vi "Find Differences.vi"() -> ()   [LabVIEW 2020]
uses:
  3e53e974-0502-4313-b7b8-032893102bf4.vi
  <vilib>/Utility/file.llb/Read Delimited Spreadsheet (DBL).vi
  <vilib>/Comparison/Equal/Equal Functor/Equal Functor.lvclass
panel:
  out "FrontDelta":dbl
  out "BackDelta":dbl
  out "Redact Data":dbl[][](graph)
  out "Org Data":dbl[][](graph)
  in  "Path":path=path "C:/Amira Data/Strip/Surface_120921_135218.csv"
  # "Average differences between close (compress) and open (decompress)"
  # "(After purging degrading data and 0s)"
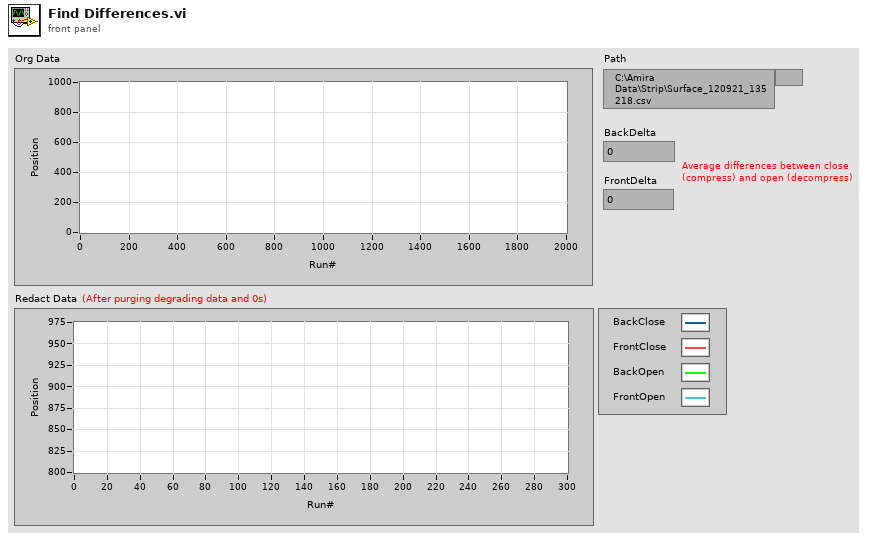
[diagram p1: front panel]
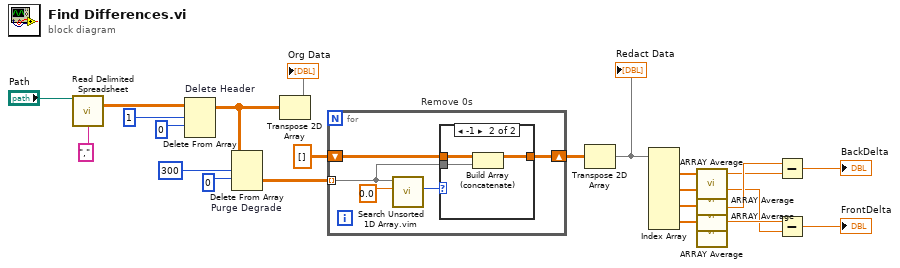
[diagram p0: block diagram]
diagram:
  n1 = call-poly <vilib>:"Read Delimited Spreadsheet.vi"("file path (dialog if empty)"="Path", "delimiter (\\t)"="," ("delimiter (\\t)")) -> ("all rows"=w21:dbl[][])  [unwired: 8 in, 5 out]
  n2 = Delete From Array "Delete Header"(array=w21, length=1, index (row)=0) -> (array with subset deleted=w17:dbl[][])  [unwired: 1 in, 1 out]
  n3 = Delete From Array "Purge Degrade"(array=w17, length=300, index (row)=0) -> (deleted portion=w14:dbl[][])  [unwired: 1 in, 1 out]
  n4 = Transpose 2D Array(2D array=w17) -> (transposed array=→"Org Data":dbl[][])
  n5 = for "Remove 0s" {
    tunnel: w14 -> [w24] mode=indexing
    shift-right: [w25] -> w12
    shift-left: dbl[][] [] -> [w26]
    n6 = call "Search Unsorted 1D Array.vim"("element"=0.0, "unsorted 1D array"=w24) -> ("index of element"=w27:i32)  [unwired: 9 in]
    n7 = case shown="-1" w27 {
      tunnel: w26 -> [w29 w32]
      tunnel: [w29 w31] -> w25
      tunnel: w24 -> [_ w30]
      frame 0, Default {
      }
      frame -1 {
        n8 = Build Array (concatenate)(w32, w30) -> (w31:dbl[][])
      }
    }
  }
  n9 = Transpose 2D Array(2D array=w12) -> (transposed array=w11:dbl[][])
  "Redact Data" <- w11
  n10 = Index Array(array=w11) -> (element #1=w10:dbl[], element #2=w9:dbl[], element #3=w8:dbl[], element #4=w7:dbl[])  [unwired: 8 in]
  n11 = call <userlib>:"ARRAY Average.vi"("Array"=w10) -> ("Ave"=w5:dbl)  [unwired: 4 in]
  n12 = call <userlib>:"ARRAY Average.vi"("Array"=w9) -> ("Ave"=w3:dbl)  [unwired: 4 in]
  n13 = call <userlib>:"ARRAY Average.vi"("Array"=w8) -> ("Ave"=w6:dbl)  [unwired: 4 in]
  n14 = call <userlib>:"ARRAY Average.vi"("Array"=w7) -> ("Ave"=w4:dbl)  [unwired: 4 in]
  n15 = Subtract(x=w6, y=w5) -> (x-y=→"BackDelta":dbl)
  n16 = Subtract(x=w4, y=w3) -> (x-y=→"FrontDelta":dbl)
